vi "tearDown.vi"(8 "error in (no error)":errorcluster, 11 "reference in":refnum<class "Test Status Updater.lvclass">) -> (0 "error out":errorcluster, 3 "reference out":refnum<class "Test Status Updater.lvclass">)   [LabVIEW 2014, in "Test Status Updater.lvclass"]
doc: "tearDown runs after the test method has completed. Use this method to clean up any operations or references that were opened by setUp or the test method. Unit tests should be independent of other unit tests so this VI should ensure that the next test can run in a 'clean' test environment."
uses:
  Test Status Updater.lvclass
  Test Status Updater.lvclass/Test Status Updater.ctl
  Core/LabVIEW CI Service/Classes/Status Updater/Status Updater.lvclass
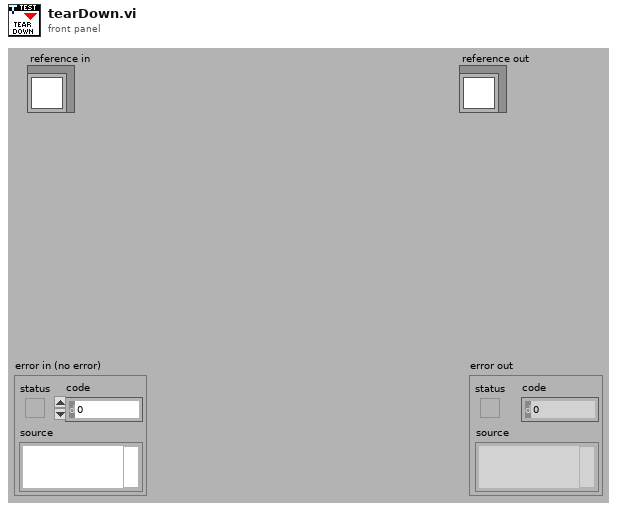
[diagram p1: front panel]
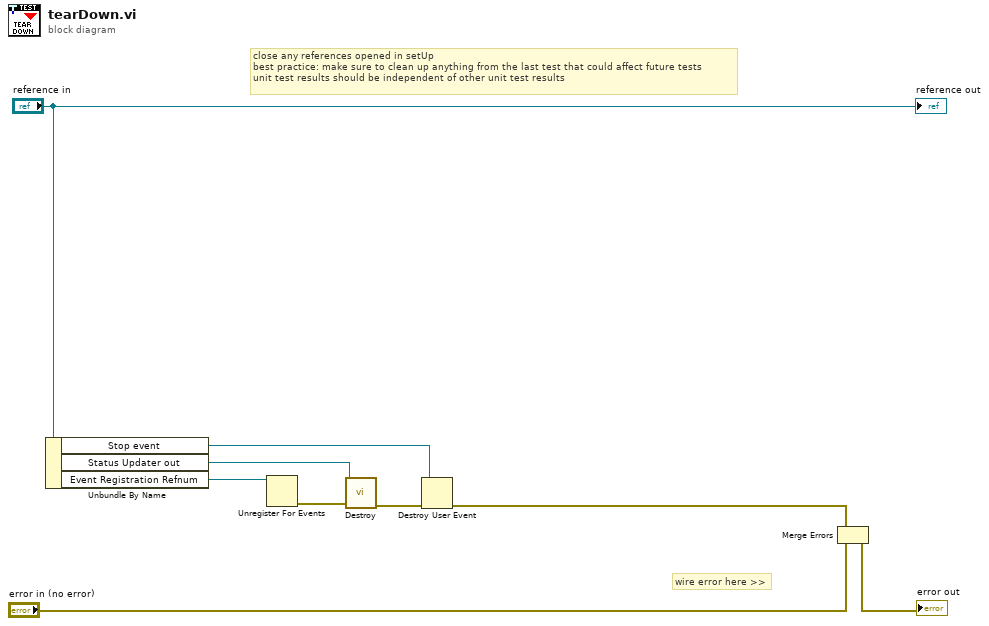
[diagram p0: block diagram]
diagram:
  # "wire error here >>"
  # "close any references opened in setUp\nbest practice: make sure to clean up anything from the last test that could affect future tests\nunit test results should be independent of other unit test results"
  n1 = Unbundle By Name("reference in") -> ("Stop event"=w2:refnum<user-event>, "Status Updater out"=w5:refnum<class "Status Updater.lvclass">, "Event Registration Refnum"=w6:refnum<event-registration>)
  n2 = Unregister For Events(event registration refnum=w6) -> (error out=w4:errorcluster)  [unwired: 1 in]
  n3 = call "Destroy.vi"("error in (no error)"=w4, "Status Updater in"=w5) -> ("error out"=w3:errorcluster)  [unwired: 9 in]
  n4 = Destroy User Event(user event=w2, error in=w3) -> (error out=w1:errorcluster)
  n5 = Merge Errors(w1, "error in (no error)") -> (→"error out":errorcluster)
  "reference out" <- "reference in"
